vi "pressurama.vi"() -> ()   [LabVIEW 2020]
uses:
  <vilib>/Instr/_visa.llb/VISA Configure Serial Port (Instr).vi
panel:
  out "Waveform Chart":cluster{dbl, dbl, dbl, dbl, dbl, dbl, dbl, dbl}(graph)={17.4, 17.3, 17.4, 17.5, 17.7, 17.6, 17.5, 17.3}
  out "x = y?":bool=TRUE
  out "trimmed string":string="0:17.40 1:17.30 2:17.40 3:17.50 4:17.70 5:17.60 6:17.50 7:17.30"
  out "number of replacements":i32=7
  in  "stop":bool
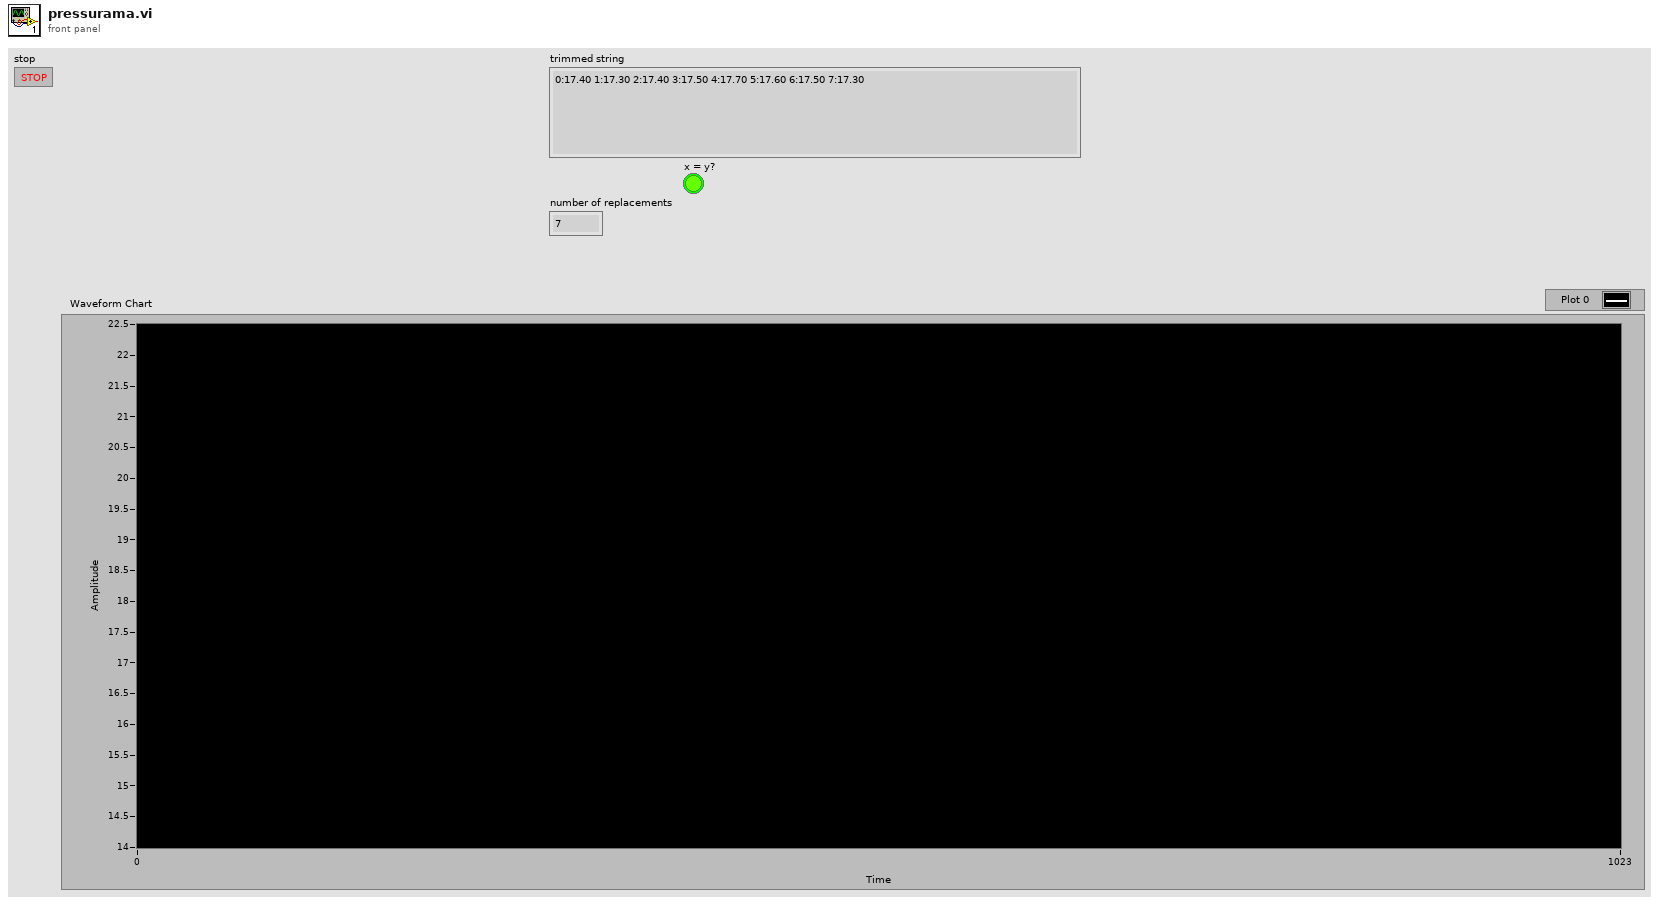
[diagram p1: front panel]
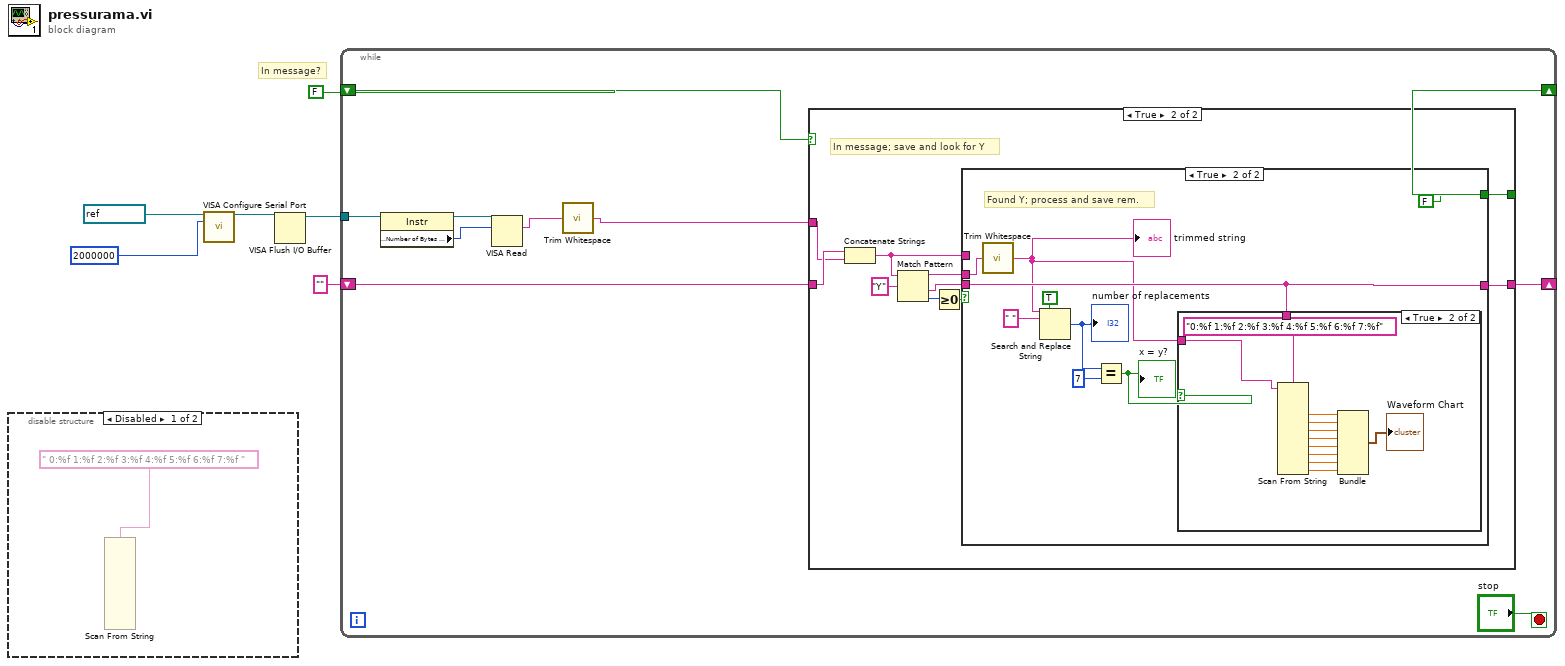
[diagram p0: block diagram]
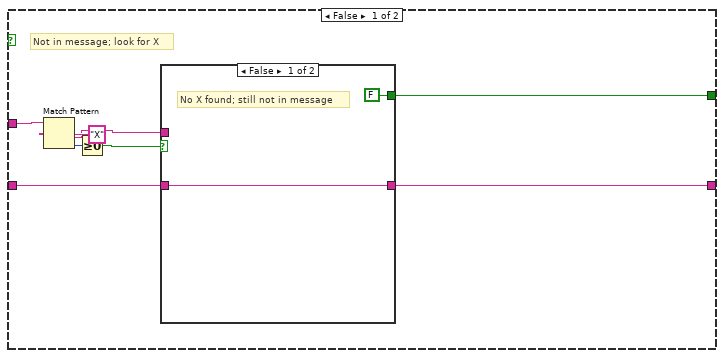
[diagram p3: hidden frame]
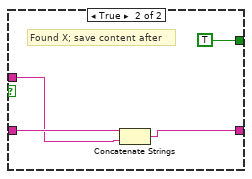
[diagram p4: hidden frame]
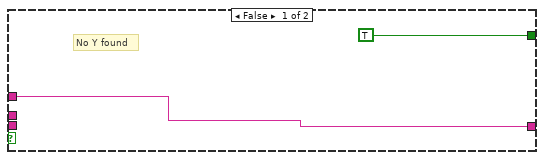
[diagram p5: hidden frame]
diagram:
  # "In message?"
  n1 = disable-structure shown="Disabled" {
    frame Disabled {
      n2 = Scan From String(format string=" 0:%f 1:%f 2:%f 3:%f 4:%f 5:%f 6:%f 7:%f ") -> ()  [unwired: 19 in, 3 out]
    }
    frame Enabled {
    }
  }
  n3 = call-poly "VISA Configure Serial Port"("VISA resource name"=refnum<visa-resource-name> "COM3", "baud rate (9600)"=u32 2000000) -> ("VISA resource name out"=w4:refnum<visa-resource-name>)  [unwired: 12 in, 1 out]
  n4 = VISA Flush I/O Buffer(VISA resource name=w4) -> (VISA resource name out=w3:refnum<visa-resource-name>)  [unwired: 2 in, 1 out]
  n5 = while {
    tunnel: w3 -> [w16]
    shift-right: [w10] -> _
    shift-left: "" -> [w12]
    shift-right: [w11] -> _
    shift-left: FALSE -> [w13]
    stop <- "stop" stop-if-true
    n6 = property class="Instr"(reference=w16) -> (reference out=w15:refnum<visa-resource-name>, "Serial Settings:Number of Bytes at Serial Port"=w14:u32)  [unwired: 1 in, 1 out]
    n7 = VISA Read(VISA resource name=w15, byte count=w14) -> (read buffer=w9:string)  [unwired: 1 in, 3 out]
    n8 = call <vilib>:"Trim Whitespace.vi"("string"=w9) -> ("trimmed string"=w8:string)  [unwired: 1 in]
    n9 = case shown="True" w13 {
      tunnel: w8 -> [w25 w40]
      tunnel: w12 -> [w20 w41]
      tunnel: [w19 w32] -> w11
      tunnel: [w18 w34] -> w10
      frame False {
        # "Not in message; look for X"
        n10 = Match Pattern(string=w25, regular expression="X") -> (after substring=w21:string, offset past match=w23:i32)  [unwired: 1 in, 2 out]
        n11 = Greater Or Equal To 0?(x=w23) -> (x >= 0?=w22:bool)
        n12 = case shown="False" w22 {
          tunnel: w21 -> [_ w30]
          tunnel: w20 -> [w26 w31]
          tunnel: [FALSE TRUE] -> w19
          tunnel: [w26 w28] -> w18
          frame False {
            # "No X found; still not in message"
          }
          frame True {
            # "Found X; save content after"
            n13 = Concatenate Strings(w31, w30) -> (w28:string)
          }
        }
      }
      frame True {
        # "In message; save and look for Y"
        n14 = Concatenate Strings(w41, w40) -> (w33:string)
        n15 = Match Pattern(string=w33, regular expression="Y") -> (before substring=w36:string, after substring=w35:string, offset past match=w39:i32)  [unwired: 1 in, 1 out]
        n16 = Greater Or Equal To 0?(x=w39) -> (x >= 0?=w37:bool)
        n17 = case shown="True" w37 {
          tunnel: w36 -> [_ w50]
          tunnel: [w43 w45] -> w34
          tunnel: w35 -> [_ w45]
          tunnel: w33 -> [w43 _]
          tunnel: [TRUE FALSE] -> w32
          frame False {
            # "No Y found"
          }
          frame True {
            # "Found Y; process and save rem."
            n18 = call <vilib>:"Trim Whitespace.vi"("string"=w50) -> ("trimmed string"=w44:string)  [unwired: 1 in]
            "trimmed string" <- w44
            n19 = Search and Replace String(replace all?=TRUE ("replace all? (F)"), input string=w44, search string=" ") -> (number of replacements=w48:i32)  [unwired: 5 in, 3 out]
            "number of replacements" <- w48
            n20 = Equal?(x=w48, y=7) -> (x = y?=w46:bool)
            "x = y?" <- w46
            n21 = case shown="True" w46 {
              tunnel: w45 -> [_ _]
              tunnel: w44 -> [_ w62]
              frame False {
              }
              frame True {
                n22 = Scan From String(format string="0:%f 1:%f 2:%f 3:%f 4:%f 5:%f 6:%f 7:%f", input string=w62) -> (output 1=w61:dbl, output 2=w54:dbl, output 3=w55:dbl, output 4=w56:dbl, output 5=w57:dbl, output 6=w58:dbl, output 7=w59:dbl, output 8=w60:dbl)  [unwired: 10 in, 3 out]
                n23 = Bundle(w61, w54, w55, w56, w57, w58, w59, w60) -> (→"Waveform Chart":cluster{dbl, dbl, dbl, dbl, dbl, dbl, dbl, dbl})  [unwired: 1 in]
              }
            }
          }
        }
      }
    }
  }
